vi "Digital Oscilloscope.vi"() -> ()   [LabVIEW 2015]
panel:
  out "error out":errorcluster
  in  "Digitizing Parameters":T1
  out "Waveform Graph":dynamicdata(graph)
  in  "stop":bool
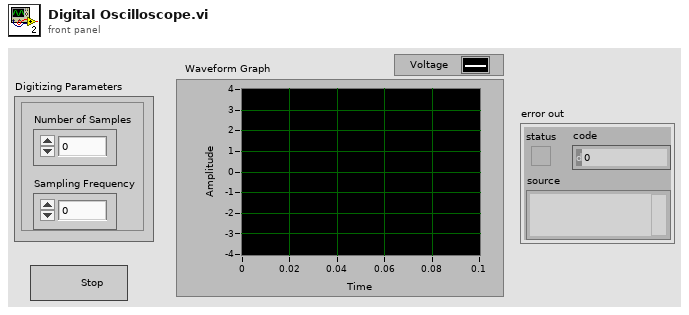
[diagram p1: front panel]
types:
  T1 = cluster{"Number of Samples":i32, "Sampling Frequency":dbl}
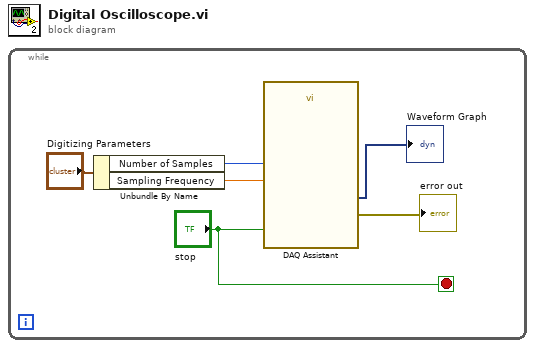
[diagram p0: block diagram]
diagram:
  n1 = while {
    stop <- "stop" stop-if-true
    n2 = Unbundle By Name("Digitizing Parameters") -> ("Number of Samples"=w5:i32, "Sampling Frequency"=w4:dbl)
    n3 = call "DAQ Assistant"("rate"=w4, "number of samples"=w5, "stop (T)"="stop") -> ("data"=→"Waveform Graph":dynamicdata, "error out"=→"error out":errorcluster)  [unwired: 14 in, 1 out]
  }
